vi "Send Current Limit.vi"(8 "error in":errorcluster, 11 "89XX in":refnum<class "89XX.lvclass">) -> (0 "error out":errorcluster, 3 "89XX out":refnum<class "89XX.lvclass">)   [LabVIEW 2019, in "89XX.lvlib" / "89XX.lvclass"]
uses:
  Library/89XX.lvclass
  C:/Users/Public/Documents/Development/builds/Instruments/PowerSupply.lvlibp/Library/PowerSupply.lvclass
  Library/89XX.lvclass/89XX.ctl
  Accessors/Read Local Resource.vi
  <instrlib>/Keysight N8900 Series/Keysight N8900 Series.lvlib
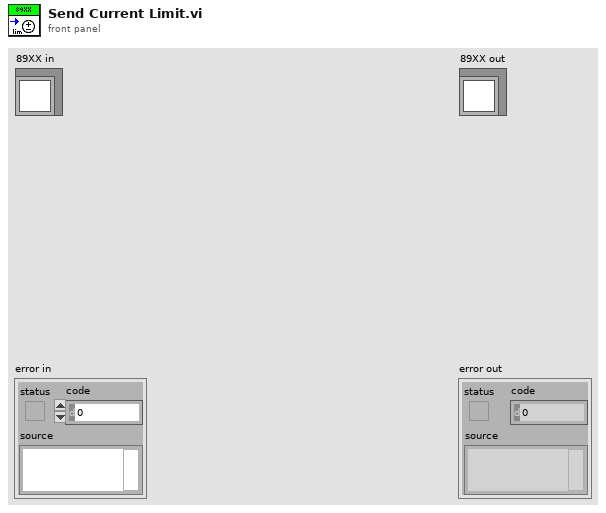
[diagram p1: front panel]
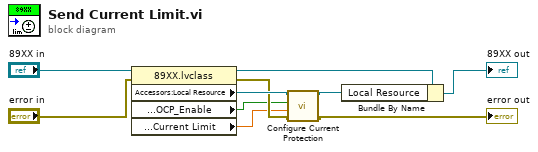
[diagram p0: block diagram]
diagram:
  n1 = property class="89XX.lvclass"(reference="89XX in", error in="error in") -> (reference out=w8:refnum<class "89XX.lvclass">, error out=w4:errorcluster, "Accessors:Local Resource"=w6:refnum<visa-resource-name>, "Accessors:Setting:Protection:OCP_Enable"=w1:bool, "Accessors:Setting:Protection:Current Limit"=w2:dbl)
  n2 = call <instrlib>:"Configure Current Protection.vi"("error in (no error)"=w4, "Protection Delay (0.05 s)"=w2, "Enable Protection (F: Disable)"=w1, "VISA resource name"=w6) -> ("error out"=→"error out":errorcluster, "VISA resource name out"=w5:refnum<visa-resource-name>)  [unwired: 6 in]
  n3 = Bundle By Name(cluster=w8, "Local Resource"=w5) -> (→"89XX out":refnum<class "89XX.lvclass">)
